vi "Basic Example.vi"() -> ()   [LabVIEW 2021]
panel:
  out "Numeric 3":dbl
  in  "Numeric 2":dbl
  in  "Numeric":dbl
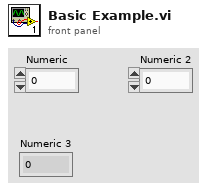
[diagram p1: front panel]
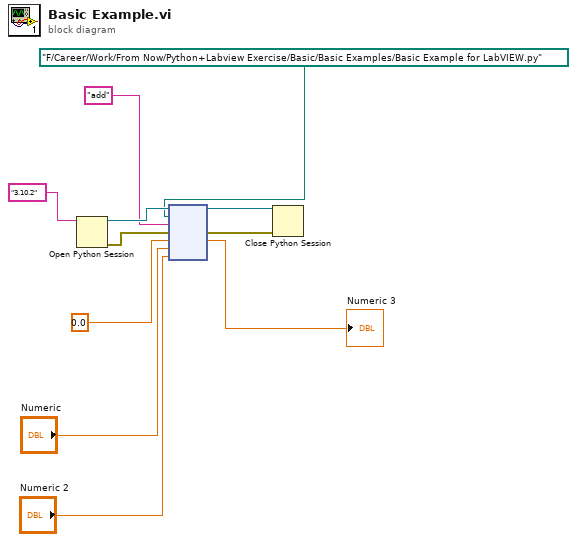
[diagram p0: block diagram]
diagram:
  n1 = Open Python Session(python version="3.10.2" ("Python version")) -> (session out=w10:refnum<k35>, error out=w7:errorcluster)  [unwired: 2 in]
  n2 = node(w10, path "F:/Career/Work/From Now/Python+Labview Exercise/Basic/Basic Examples/Basic Example for LabVIEW.py" ("module path"), "add" ("function name"), w7, 0.0, "Numeric", "Numeric 2") -> (w9:refnum<k35>, w8:errorcluster, →"Numeric 3":dbl)  [unwired: 2 in, 2 out]
  n3 = Close Python Session(session in=w9, error in=w8) -> ()  [unwired: 1 out]
